vi "unload.vi"(7 "TaskRef in":refnum<vi>, 8 "error in (no error)":errorcluster, 9 "pdbm_task_reg_reqst_event":refnum<event-registration>, 10 "pdbm_task_data":T1, 11 "pdbm_task_event":T2) -> (0 "error out":errorcluster, 3 "pdbm_taskroute_feedback_event":refnum<user-event>, 5 "TaskRef out":refnum<vi>)   [LabVIEW 2015, in "pdbm_tasks.lvlib"]
uses:
  pdbm_tasks.lvlib
  pdbm_test_route/UsrDefine/TaskReqst.ctl
  pdbm_test_route/UsrDefine/TaskFeedbackCmd.ctl
  UsrDefine/PDBM_TestSystem_Data.ctl
  pdbm_test_route/pdbm_task_route.lvlib
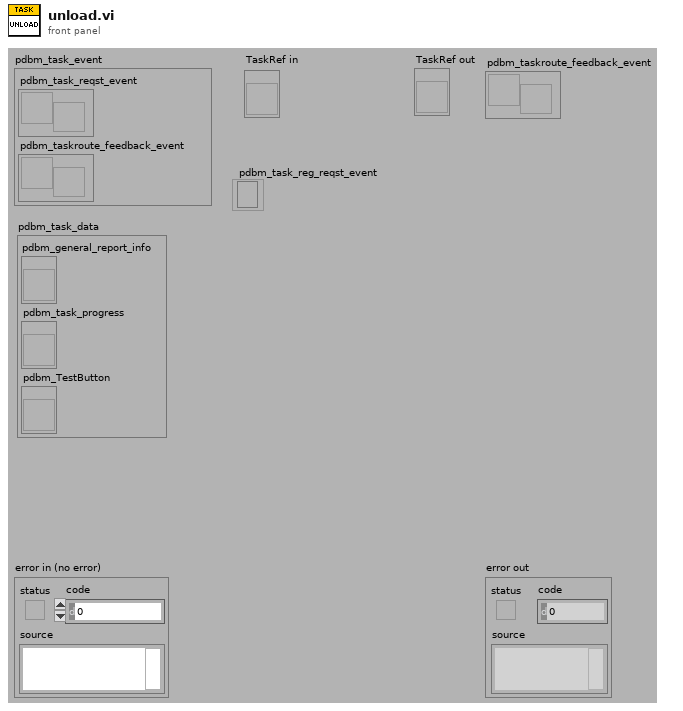
[diagram p1: front panel]
types:
  T1 = typedef "pdbm_tasks.lvlib/PDBM_TestSystem_Data.ctl" = cluster{"pdbm_general_report_info":refnum<vi>, "pdbm_task_progress":refnum<vi>, "pdbm_TestButton":refnum<vi>}
  T2 = cluster{"pdbm_task_reqst_event":refnum<user-event>, "pdbm_taskroute_feedback_event":refnum<user-event>}
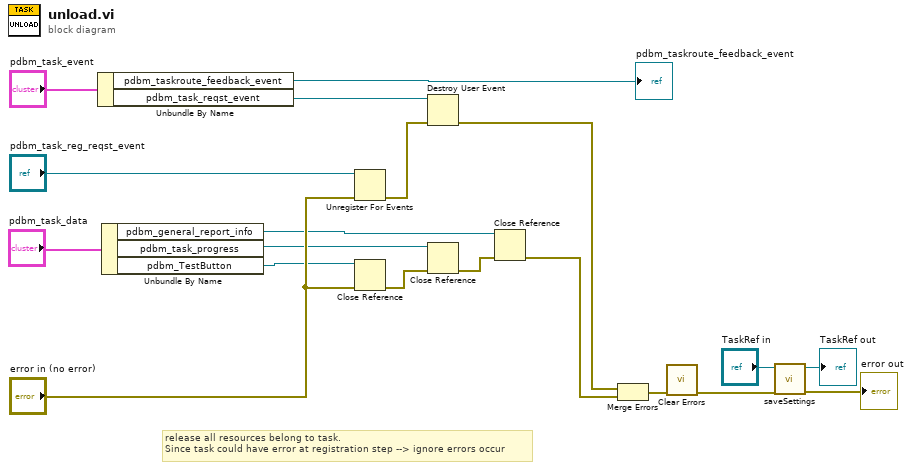
[diagram p0: block diagram]
diagram:
  # "release all resources belong to task.\nSince task could have error at registration step --> ignore errors occur"
  n1 = Unbundle By Name("pdbm_task_event") -> ("pdbm_taskroute_feedback_event"=→"pdbm_taskroute_feedback_event":refnum<user-event>, "pdbm_task_reqst_event"=w16:refnum<user-event>)
  n2 = Unbundle By Name("pdbm_task_data") -> ("pdbm_general_report_info"=w7:refnum<vi>, "pdbm_task_progress"=w8:refnum<vi>, "pdbm_TestButton"=w9:refnum<vi>)
  n3 = Unregister For Events(event registration refnum="pdbm_task_reg_reqst_event", error in="error in (no error)") -> (error out=w15:errorcluster)
  n4 = Close Reference(reference=w9, error in (no error)="error in (no error)") -> (error out=w11:errorcluster)
  n5 = Destroy User Event(user event=w16, error in=w15) -> (error out=w12:errorcluster)
  n6 = Close Reference(reference=w8, error in (no error)=w11) -> (error out=w6:errorcluster)
  n7 = Close Reference(reference=w7, error in (no error)=w6) -> (error out=w5:errorcluster)
  n8 = Merge Errors(w12, w5) -> (w13:errorcluster)
  n9 = call <vilib>:"Clear Errors.vi"("error in (no error)"=w13) -> ("error out"=w4:errorcluster)  [unwired: 5 in, 1 out]
  n10 = call "saveSettings.vi"("error in (no error)"=w4, "TaskRef in"="TaskRef in") -> ("error out"=→"error out":errorcluster, "TaskRef out"=→"TaskRef out":refnum<vi>)  [unwired: 8 in]
